vi "Cleanup.vi"(8 "error in (no error)":errorcluster, 11 "Channel in":refnum<class "Channel.lvclass">) -> (0 "error out":errorcluster)   [LabVIEW 2019, in "Channel.lvclass"]
uses:
  Channel.lvclass
  Channel.lvclass/Channel.ctl
  Effect/Effect.lvclass
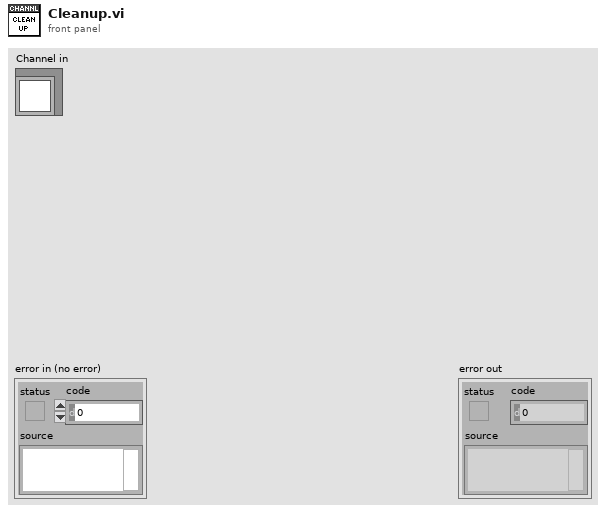
[diagram p1: front panel]
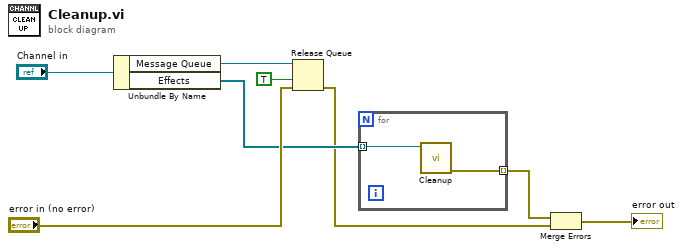
[diagram p0: block diagram]
diagram:
  n1 = Unbundle By Name("Channel in") -> ("Message Queue"=w5:refnum<queue>, "Effects"=w4:refnum<class "Effect.lvclass">[])
  n2 = Release Queue(queue=w5, force destroy? (F)=TRUE, error in (no error)="error in (no error)") -> (error out=w1:errorcluster)  [unwired: 2 out]
  n3 = for {
    tunnel: w4 -> [w10] mode=indexing
    tunnel: [w9] -> w3 mode=indexing
    n4 = call "Cleanup.vi"("Effect in"=w10) -> ("error out"=w9:errorcluster)  [unwired: 10 in]
  }
  n5 = Merge Errors(w3, w1) -> (→"error out":errorcluster)
